vi "SHA-1 Core.vi"(0 "s1":u32=1732584193 format="%.0x", 1 "Input Bytes":u8[](array[numeric]), 5 "s2":u32=4023233417 format="%.0x", 7 "s3":u32=2562383102 format="%.0x", 9 "s4":u32=271733878 format="%.0x", 11 "s5":u32=271733878 format="%.0x") -> (4 "s1 out":u32, 6 "s2 out":u32, 8 "s3 out":u32, 10 "s4 out":u32, 15 "s5 out":u32)   [LabVIEW 2016, in "websocket core.lvlib"]
doc: "This VI contains the core of the MD5 algorithm."
uses:
  websocket core.lvlib
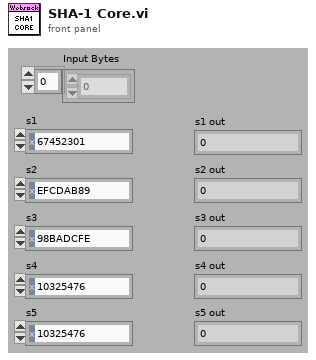
[diagram p1: front panel]
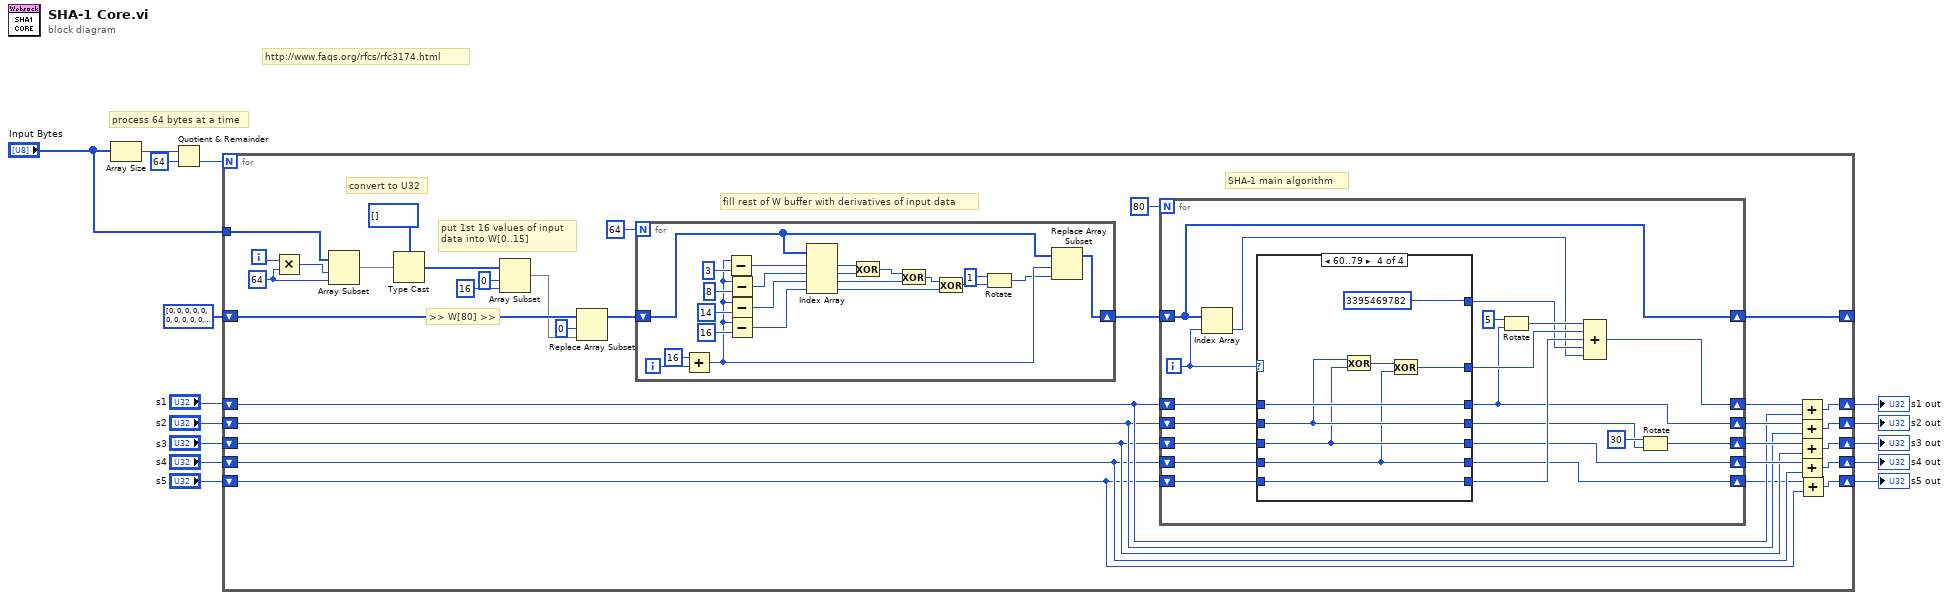
[diagram p0: block diagram]
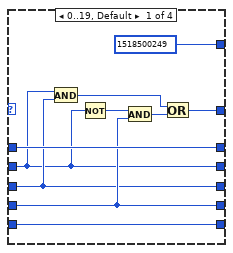
[diagram p2: hidden frame]
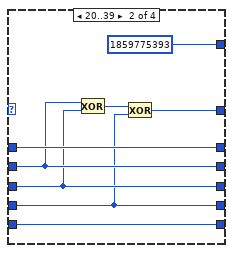
[diagram p3: hidden frame]
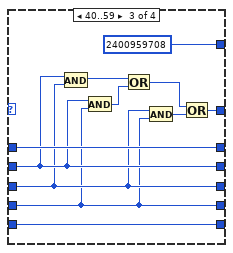
[diagram p4: hidden frame]
diagram:
  # "process 64 bytes at a time"
  # "http://www.faqs.org/rfcs/rfc3174.html"
  n1 = Array Size(array="Input Bytes") -> (size(s)=w3:i32)
  n2 = Quotient & Remainder(x=w3, y=64) -> (floor(x/y)=w15:i32)  [unwired: 1 out]
  n3 = for {
    N: w15 -> [_]
    shift-right: [w43] -> w13
    shift-left: "s1" -> [w39]
    shift-right: [w42] -> w12
    shift-left: "s2" -> [w38]
    shift-right: [w41] -> w11
    shift-left: "s3" -> [w37]
    shift-right: [w40] -> w10
    shift-left: "s4" -> [w36]
    tunnel: "Input Bytes" -> [w32]
    shift-right: [w33] -> w4
    shift-left: "s5" -> [w29]
    shift-right: [w20] -> _
    shift-left: u32[] [0, 0, 0, 0, 0, 0, 0, 0, 0, 0, 0, 0, 0, 0, 0, 0, 0, 0, 0, 0, 0, 0, 0, 0, 0, 0, 0, 0, 0, 0, 0, 0, 0, 0, 0, 0, 0, 0, 0, 0, 0, 0, 0, 0, 0, 0, 0, 0, 0, 0, 0, 0, 0, 0, 0, 0, 0, 0, 0, 0, 0, 0, 0, 0, 0, 0, 0, 0, 0, 0, 0, 0, 0, 0, 0, 0, 0, 0, 0, 0] -> [w25]
    i -> [w35]
    w31 = 64 ("y")
    # "SHA-1 main algorithm"
    # "fill rest of W buffer with derivatives of input data"
    # ">> W[80] >>"
    # "put 1st 16 values of input data into W[0..15]"
    # "convert to U32"
    n4 = Multiply(x=w35, y=w31) -> (x*y=w30:i32)
    n5 = Array Subset(array=w32, index=w30, length=w31) -> (w27:u8[])
    n6 = Type Cast(type=u32[] [], x=w27) -> (*(type *) &x=w26:u32[])
    n7 = Array Subset(array=w26, index=0, length=16) -> (w19:u32[])
    n8 = Replace Array Subset(array=w25, new element=w19, index=0) -> (w24:u32[])
    n9 = for {
      N: 64 -> [_]
      shift-right: [w116] -> w21
      shift-left: w24 -> [w114]
      i -> [w126]
      n10 = Add(x=16, y=w126) -> (x+y=w115:i32)
      n11 = Subtract(x=w115, y=3) -> (x-y=w122:i32)
      n12 = Subtract(x=w115, y=8) -> (x-y=w119:i32)
      n13 = Subtract(x=w115, y=14) -> (x-y=w118:i32)
      n14 = Subtract(x=w115, y=16) -> (x-y=w117:i32)
      n15 = Index Array(array=w114, index #1=w122, index #2=w119, index #3=w118, index #4=w117) -> (element #1=w113:u32, element #2=w112:u32, element #3=w110:u32, element #4=w108:u32)
      n16 = Exclusive Or(1:w112, 2:w113) -> (0:w111:u32)
      n17 = Exclusive Or(1:w110, 2:w111) -> (0:w109:u32)
      n18 = Exclusive Or(1:w108, 2:w109) -> (0:w107:u32)
      n19 = Rotate(1:w107, 2:i8 1 ("y")) -> (0:w106:u32)
      n20 = Replace Array Subset(array=w114, new element=w106, index=w115) -> (w116:u32[])
    }
    n21 = for {
      N: 80 -> [_]
      shift-right: [w55] -> w44
      shift-left: w39 -> [w67]
      shift-right: [w54] -> w45
      shift-left: w38 -> [w66]
      shift-right: [w51] -> w46
      shift-left: w37 -> [w65]
      shift-right: [w50] -> w47
      shift-left: w36 -> [w64]
      shift-right: [w49] -> w34
      shift-left: w29 -> [w63]
      shift-right: [w48] -> w20
      shift-left: w21 -> [w48]
      i -> [w57]
      n22 = Index Array(array=w48, index=w57) -> (element=w56:u32)
      n23 = case shown="60..79" w57 {
        tunnel: w67 -> [w72 w85 w96 w103]
        tunnel: w66 -> [w68 w82 w91 w99]
        tunnel: w65 -> [w69 w81 w87 w98]
        tunnel: w64 -> [w71 w79 w86 w97]
        tunnel: w63 -> [w70 w84 w95 w102]
        tunnel: [w72 w85 w96 w103] -> w54
        tunnel: [w68 w82 w91 w99] -> w52
        tunnel: [w69 w81 w87 w98] -> w50
        tunnel: [w71 w79 w86 w97] -> w49
        tunnel: [w70 w84 w95 w102] -> w59
        tunnel: [w74 w78 w88 w100] -> w60
        tunnel: [u32 1518500249 u32 1859775393 u32 2400959708 u32 3395469782] -> w58
        frame 0..19, Default {
          n24 = And(x=w68, y=w69) -> (x .and. y?=w75:u32)
          n25 = Not(x=w68) -> (.not. x?=w77:u32)
          n26 = And(x=w77, y=w71) -> (x .and. y?=w76:u32)
          n27 = Or(x=w75, y=w76) -> (x .or. y?=w74:u32)
        }
        frame 20..39 {
          n28 = Exclusive Or(1:w81, 2:w82) -> (0:w80:u32)
          n29 = Exclusive Or(1:w79, 2:w80) -> (0:w78:u32)
        }
        frame 40..59 {
          n30 = And(x=w91, y=w87) -> (x .and. y?=w92:u32)
          n31 = And(x=w91, y=w86) -> (x .and. y?=w93:u32)
          n32 = Or(x=w92, y=w93) -> (x .or. y?=w90:u32)
          n33 = And(x=w87, y=w86) -> (x .and. y?=w89:u32)
          n34 = Or(x=w90, y=w89) -> (x .or. y?=w88:u32)
        }
        frame 60..79 {
          n35 = Exclusive Or(1:w98, 2:w99) -> (0:w101:u32)
          n36 = Exclusive Or(1:w97, 2:w101) -> (0:w100:u32)
        }
      }
      n37 = Rotate(1:w54, 2:i8 5 ("y")) -> (0:w61:u32)
      n38 = Compound Arithmetic op=ADD(w61, w60, w59, w58, w56) -> (w55:u32)
      n39 = Rotate(1:w52, 2:i8 30 ("y")) -> (0:w51:u32)
    }
    n40 = Add(x=w44, y=w39) -> (x+y=w43:u32)
    n41 = Add(x=w45, y=w38) -> (x+y=w42:u32)
    n42 = Add(x=w46, y=w37) -> (x+y=w41:u32)
    n43 = Add(x=w47, y=w36) -> (x+y=w40:u32)
    n44 = Add(x=w34, y=w29) -> (x+y=w33:u32)
  }
  "s1 out" <- w13
  "s2 out" <- w12
  "s3 out" <- w11
  "s4 out" <- w10
  "s5 out" <- w4
